vi "Local Joint Reference Follower.vi"(6 "Digital Cmd [0-78]":i8, 7 "Offset Home2RCM [deg/mm]":dbl[](array[numeric])=[0.0, 0.0, 0.0, 0.0], 8 "PID Ctrl Cluster":T1={"L1 PID Gains"={"Kp"=0.005, "Kd"=0.5, "Ki"=0.0005}, "L2 PID Gains"={"Kp"=0.01, "Kd"=1.0, "Ki"=0.005}, "L3 PID Gains"={"Kp"=0.05, "Kd"=1.0, "Ki"=0.0005}, "L4 PID Gains"={"Kp"=0.1, "Kd"=0.1, "Ki"=0.0005}}, 9 "Ref Array [deg/mm]":dbl[](array[numeric])=[0.0, 0.0, 0.0, 0.0], 10 "error in":errorcluster, 11 "FPGA VI Reference In":refnum<k20>) -> (1 "Output Posit Array [deg/mm]":dbl[](array[numeric]), 2 "error out":errorcluster, 3 "FPGA VI Reference Out":refnum<k20>)   [LabVIEW 2016]
uses:
  <vilib>/rvi/errors/niLvFpgaAdjustHostInterfaceError.vi
  <vilib>/Utility/error.llb/Error Cluster From Error Code.vi
  Subsystems/Global Variables.vi
  <vilib>/rvi/interface/nirviReadWriteControl/nirviReadWriteControl.xnode
  FPGA Bitfiles/PhantomControlPI_FPGATarget_QuadCtr2_E2412E44.lvbitx
  IRISS_FPGA_IO.vi
  Library/KevinLibraryAll/labview/KevLib01.lvlib
  NiFpgaLv.dll
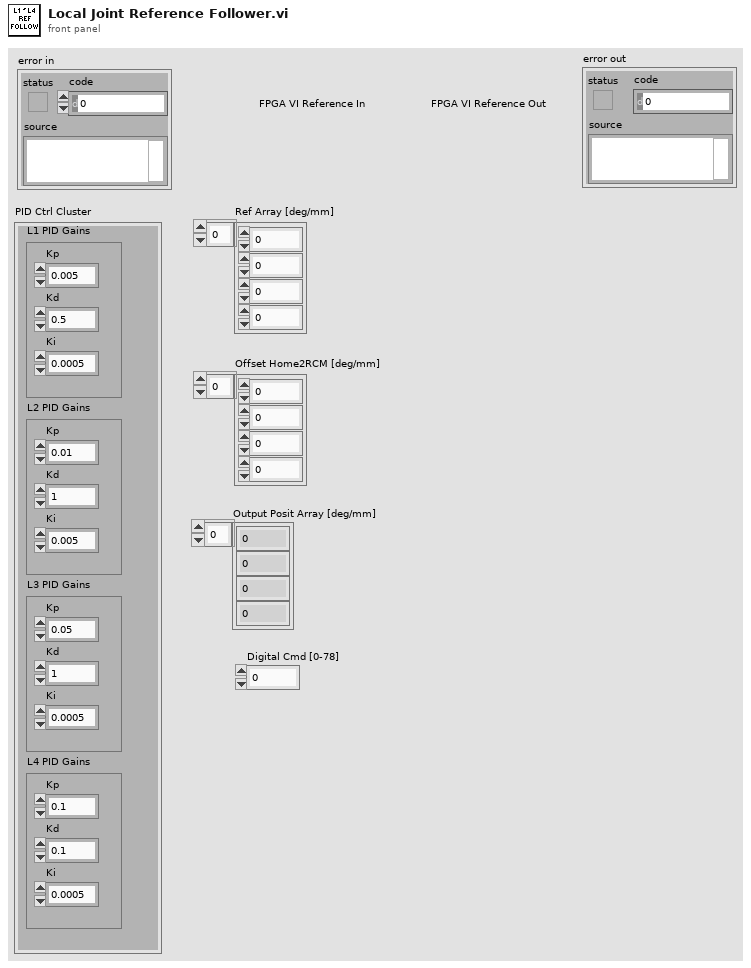
[diagram p1: front panel]
types:
  T1 = cluster{"L1 PID Gains":cluster{"Kp":dbl, "Kd":dbl, "Ki":dbl}, "L2 PID Gains":cluster{"Kp":dbl, "Kd":dbl, "Ki":dbl}, "L3 PID Gains":cluster{"Kp":dbl, "Kd":dbl, "Ki":dbl}, "L4 PID Gains":cluster{"Kp":dbl, "Kd":dbl, "Ki":dbl}}
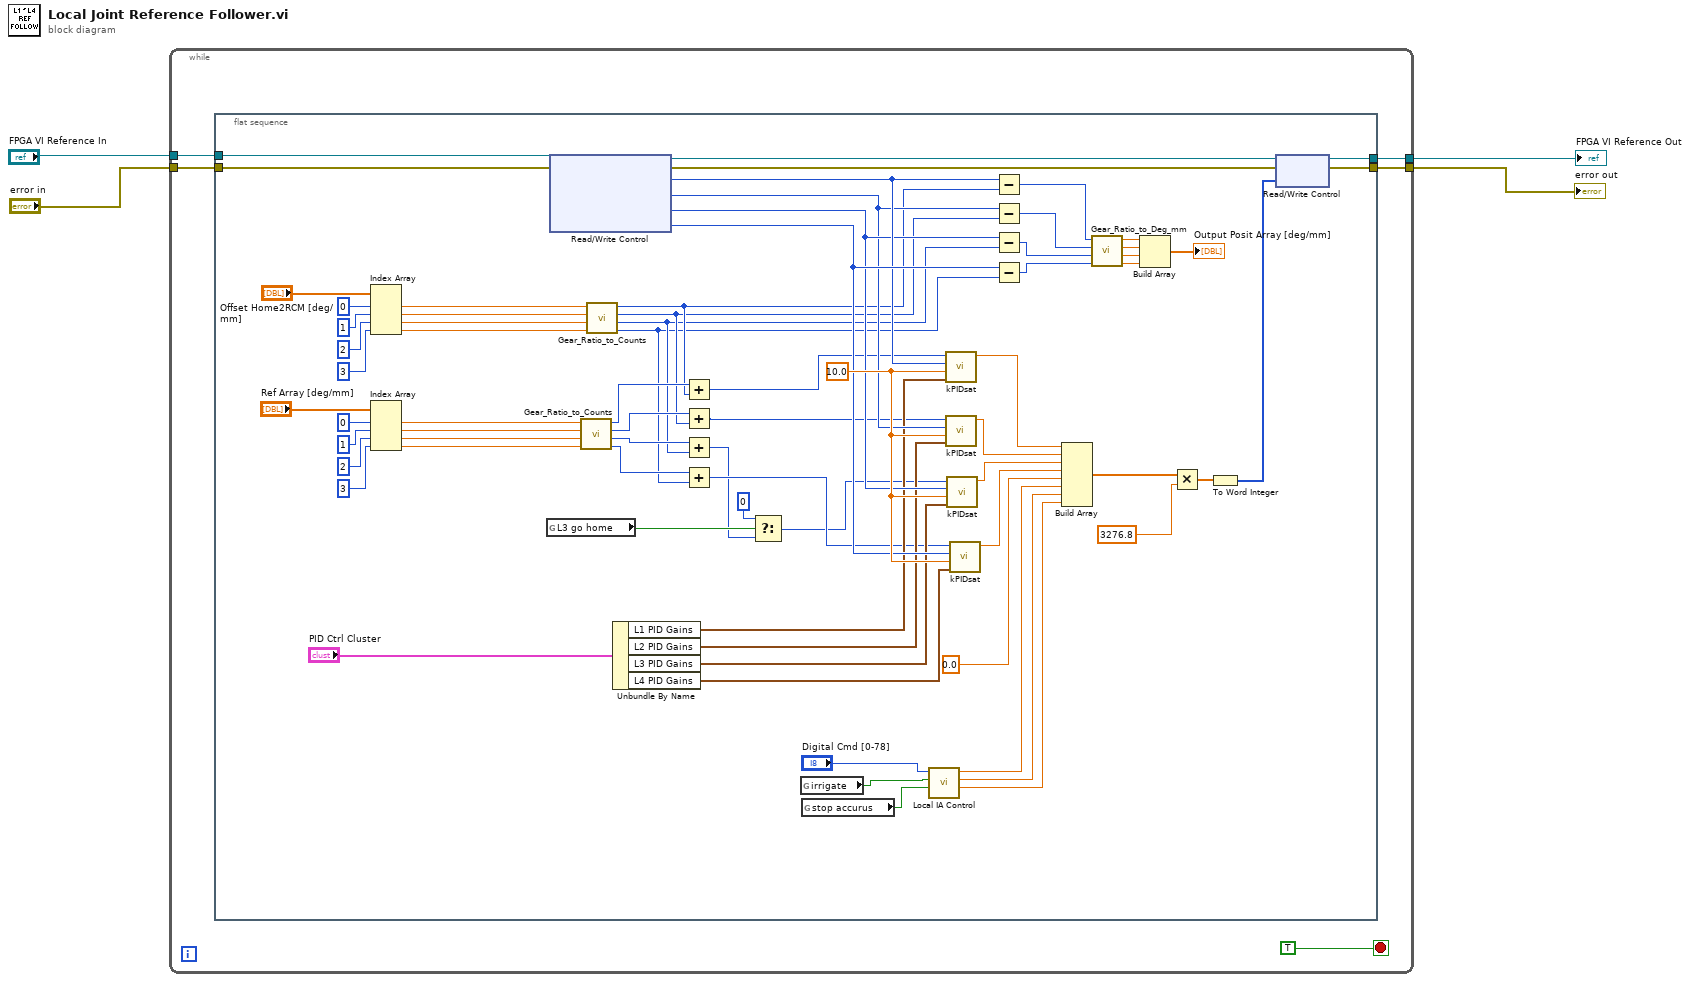
[diagram p0: block diagram]
diagram:
  n1 = while {
    tunnel: [w9] -> w1
    tunnel: [w8] -> w4
    tunnel: "FPGA VI Reference In" -> [w7]
    tunnel: "error in" -> [w6]
    stop <- TRUE ("Boolean") stop-if-true
    n2 = flat-sequence {
      tunnel: [w61] -> w9
      tunnel: [w60] -> w8
      tunnel: w7 -> [w38]
      tunnel: w6 -> [w37]
      frame #0 {
        w68 = 10.0 ("Sat Limit")
        n3 = Index Array(array="Offset Home2RCM [deg/mm]", index #1=0 ("index"), index #2=1 ("index"), index #3=2 ("index"), index #4=3 ("index")) -> (element #1=w36:dbl, element #2=w35:dbl, element #3=w34:dbl, element #4=w33:dbl)
        n4 = Index Array(array="Ref Array [deg/mm]", index #1=0 ("index"), index #2=1 ("index"), index #3=2 ("index"), index #4=3 ("index")) -> (element #1=w76:dbl, element #2=w75:dbl, element #3=w74:dbl, element #4=w10:dbl)
        n5 = global read "Global Variables.vi" "L3 go home"() -> (w21:bool)
        n6 = xnode "Read/Write Control"("FPGA VI Reference In"=w38, "error in"=w37) -> ("FPGA VI Reference Out"=w63:refnum<k20>, "error out"=w62:errorcluster, "32 bit Position 1"=w45:i32, "32 bit Position 3"=w43:i32, "32 bit Position C1-1"=w44:i32, "32 bit Position C1-4"=w55:i32)
        n7 = call "Gear_Ratio_to_Counts.vi"("theta 4"=w10, "theta 3"=w74, "theta 2"=w75, "theta 1"=w76) -> ("j4"=w26:i32, "j3"=w27:i32, "j2"=w28:i32, "j1"=w29:i32)
        n8 = call "Gear_Ratio_to_Counts.vi"("theta 4"=w33, "theta 3"=w34, "theta 2"=w35, "theta 1"=w36) -> ("j4"=w22:i32, "j3"=w23:i32, "j2"=w24:i32, "j1"=w25:i32)
        n9 = Unbundle By Name("PID Ctrl Cluster") -> ("L1 PID Gains"=w42:cluster{"Kp":dbl, "Kd":dbl, "Ki":dbl}, "L2 PID Gains"=w41:cluster{"Kp":dbl, "Kd":dbl, "Ki":dbl}, "L3 PID Gains"=w40:cluster{"Kp":dbl, "Kd":dbl, "Ki":dbl}, "L4 PID Gains"=w39:cluster{"Kp":dbl, "Kd":dbl, "Ki":dbl})
        n10 = Add(x=w29, y=w25) -> (x+y=w32:i32)
        n11 = Add(x=w28, y=w24) -> (x+y=w31:i32)
        n12 = Add(x=w27, y=w23) -> (x+y=w20:i32)
        n13 = Add(x=w26, y=w22) -> (x+y=w30:i32)
        n14 = Select(t=0 ("index"), s=w21, f=w20) -> (s? t:f=w18:i32)
        n15 = global read "Global Variables.vi" "irrigate"() -> (w12:bool)
        n16 = global read "Global Variables.vi" "stop accurus"() -> (w11:bool)
        n17 = call "Local IA Control.vi"("E-Stop Vacuum"=w11, "Irrigate?"=w12, "8bit integer"="Digital Cmd [0-78]") -> ("Accurus Engaged Vout"=w15:dbl, "Accurus ChB Vout"=w14:dbl, "Accurus ChA Vout"=w16:dbl)  [unwired: 6 in]
        n18 = call "kPIDsat.vi"("PID Gains"=w42, "Sat Limit"=w68, "Position"=w45, "Reference"=w32) -> ("Control"=w54:dbl)  [unwired: 7 in]
        n19 = call "kPIDsat.vi"("PID Gains"=w41, "Sat Limit"=w68, "Position"=w43, "Reference"=w31) -> ("Control"=w56:dbl)  [unwired: 7 in]
        n20 = call "kPIDsat.vi"("PID Gains"=w40, "Sat Limit"=w68, "Position"=w44, "Reference"=w18) -> ("Control"=w57:dbl)  [unwired: 7 in]
        n21 = call "kPIDsat.vi"("PID Gains"=w39, "Sat Limit"=w68, "Position"=w55, "Reference"=w30) -> ("Control"=w67:dbl)  [unwired: 7 in]
        n22 = Subtract(x=w45, y=w25) -> (x-y=w49:i32)
        n23 = Subtract(x=w43, y=w24) -> (x-y=w48:i32)
        n24 = Subtract(x=w44, y=w23) -> (x-y=w47:i32)
        n25 = Subtract(x=w55, y=w22) -> (x-y=w46:i32)
        n26 = Build Array(w54, w56, w57, w67, 0.0 ("element"), w16, w14, w15) -> (w17:dbl[])
        n27 = call "Gear_Ratio_to_Deg_mm.vi"("j4"=w46, "j3"=w47, "j2"=w48, "j1"=w49) -> ("theta 4"=w50:dbl, "theta 3"=w51:dbl, "theta 2"=w52:dbl, "theta 1"=w53:dbl)
        n28 = Build Array(w53, w52, w51, w50) -> (→"Output Posit Array [deg/mm]":dbl[])
        n29 = Multiply(x=w17, y=3276.8) -> (x*y=w65:dbl[])
        n30 = To Word Integer(number=w65) -> (16bit integer=w64:i16[])
        n31 = xnode "Read/Write Control"("FPGA VI Reference In"=w63, "error in"=w62, "AO"=w64) -> ("FPGA VI Reference Out"=w61:refnum<k20>, "error out"=w60:errorcluster)
      }
    }
  }
  "error out" <- w4
  "FPGA VI Reference Out" <- w1
